vi "15-1.vi"() -> ()   [LabVIEW 2019, in "15.lvlib"]
uses:
  15.lvlib
panel:
  in  "Sample Input?":bool
  out "Lowest Risk":u64
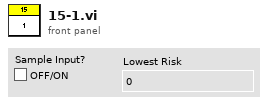
[diagram p1: front panel]
types:
  T1 = map{cluster{"Row":i32, "Col":i32}, cluster{"Adjacency Matrix":cluster{i32, i32}[], "Risk":u8, "Min Risk":i32, "Visited?":bool}}
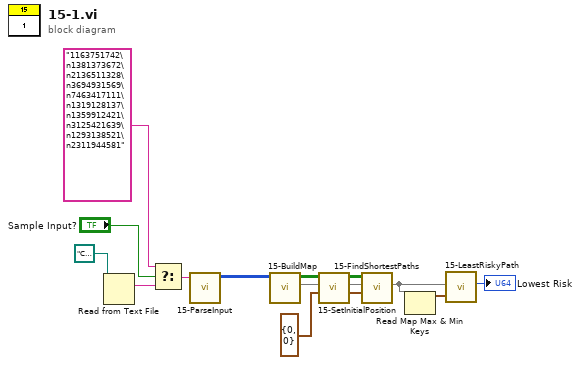
[diagram p0: block diagram]
diagram:
  n1 = Read from Text File(file (use dialog)=path "C:/Users/craig.walker/Documents/GitHub/lv2019-Advent-of-Code-2021/15/input.txt") -> (text=w10:string)  [unwired: 3 in, 3 out]
  n2 = Select(t="1163751742\n1381373672\n2136511328\n3694931569\n7463417111\n1319128137\n1359912421\n3125421639\n1293138521\n2311944581", s="Sample Input?", f=w10) -> (s? t:f=w11:string)
  n3 = call "15-ParseInput.vi"("String"=w11) -> ("Risk Array"=w1:u8[][])  [unwired: 10 in]
  n4 = call "15-BuildMap.vi"("Risk Array"=w1) -> ("map"=w12:T1, "Visited Array"=w14:bool[][])  [unwired: 9 in]
  n5 = call "15-SetInitialPosition.vi"("Initial Position in"=cluster{"Row":i32, "Col":i32} {"Row"=0, "Col"=0}, "map in"=w12, "Visited Array in"=w14) -> ("Initial Position out"=w7:cluster{"Row":i32, "Col":i32}, "map out"=w6:T1, "Visited Array out"=w13:bool[][])  [unwired: 6 in]
  n6 = call "15-FindShortestPaths.vi"("Initial Position"=w7, "map in"=w6, "Visited Array in"=w13) -> ("map out"=w4:T1)  [unwired: 8 in]
  n7 = Read Map Max & Min Keys(11:w4) -> (3:w3:cluster{"Row":i32, "Col":i32})  [unwired: 1 out]
  n8 = call "15-LeastRiskyPath.vi"("position"=w3, "map in"=w4) -> ("Min Risk"=→"Lowest Risk":i32)  [unwired: 9 in]
